vi "mainUI.vi"(8 "Error In":errorcluster, 10 "UI Data":T1, 11 "UDE Data":T14) -> (0 "Error Out":errorcluster)   [LabVIEW 2018]
uses:
  controls/uiUDE.ctl
  controls/uiData.ctl
  controls/pathCluster.ctl
  controls/shiftCluster.ctl
  controls/modelHomeCluster.ctl
  controls/hardwareSignalCluster.ctl
  controls/printedBarcodeCluster.ctl
  controls/scannedBarcode.ctl
  controls/reportCluster.ctl
  controls/modelSettingsCluster.ctl
  controls/LHndRH.ctl
  controls/ModelTableCluster.ctl
  controls/overrideCluster.ctl
  controls/countCluster.ctl
  Controller Module/src/controls/controllerData.ctl
  controls/mainAppElementsCluster.ctl
  Modbus Module/src/controls/modbusData.ctl
  controls/readRegisterModbusCluster.ctl
  Barcode Printer Module/src/controls/printData.ctl
  Barcode Scanner Module/src/controls/scanData.ctl
panel:
  out "Tab Control":enum32{"Home", "Report", "Settings"}(tab)
  out "TRACEABILITY GRAPH":cluster{"X":dbl, "Y":dbl}[](graph)
  out "PRODUCTION DATE":string
  out "SEQUENCE NUMBER":string
  out "PART NUMBER":string
  out "SUPPLIER CODE":string
  out "MODEL":string
  out "PRINTED BARCODE":cluster{"Value":string}
  out "SCANNED BARCODE":cluster{"Value":string}
  out "TOTAL":dbl
  out "NG":dbl
  out "OK":dbl
  out "SHIFT":string
  out "Scanner":bool
  out "Printer":bool
  out "Database":bool
  out "PLC":bool
  in  "Settings":bool
  in  "Report":bool
  in  "Stop":bool
  out "Application Name":string
  out "Result Table":string[][](table)
  out "Status":string
  out "Version No":string
  in  "Reprint":bool
  in  "TO DATE":timestamp format="%<%x %.3X>T"
  in  "Fetch":bool
  in  "Export":bool
  in  "FROM DATE":timestamp format="%<%x %.3X>T"
  out "Report Table":string[][](table)
  in  "Home":bool
  in  "NG":string
  in  "OK":string
  in  "SEQUENCE NUMBER":string
  in  "Override Button":bool
  in  "Load Button":bool
  in  "Home Button":bool
  in  "Delete Button":bool
  in  "Update Button":bool
  in  "Save Button":bool
  in  "PLC NUMBER":string
  in  "LH / RH":T10
  in  "SUPPLIER CODE":string
  in  "CUSTOMER PART NUMBER":string
  in  "SAVED MODEL":string(combo)
  out "Model Table":string[][](table)
  in  "MODEL":string
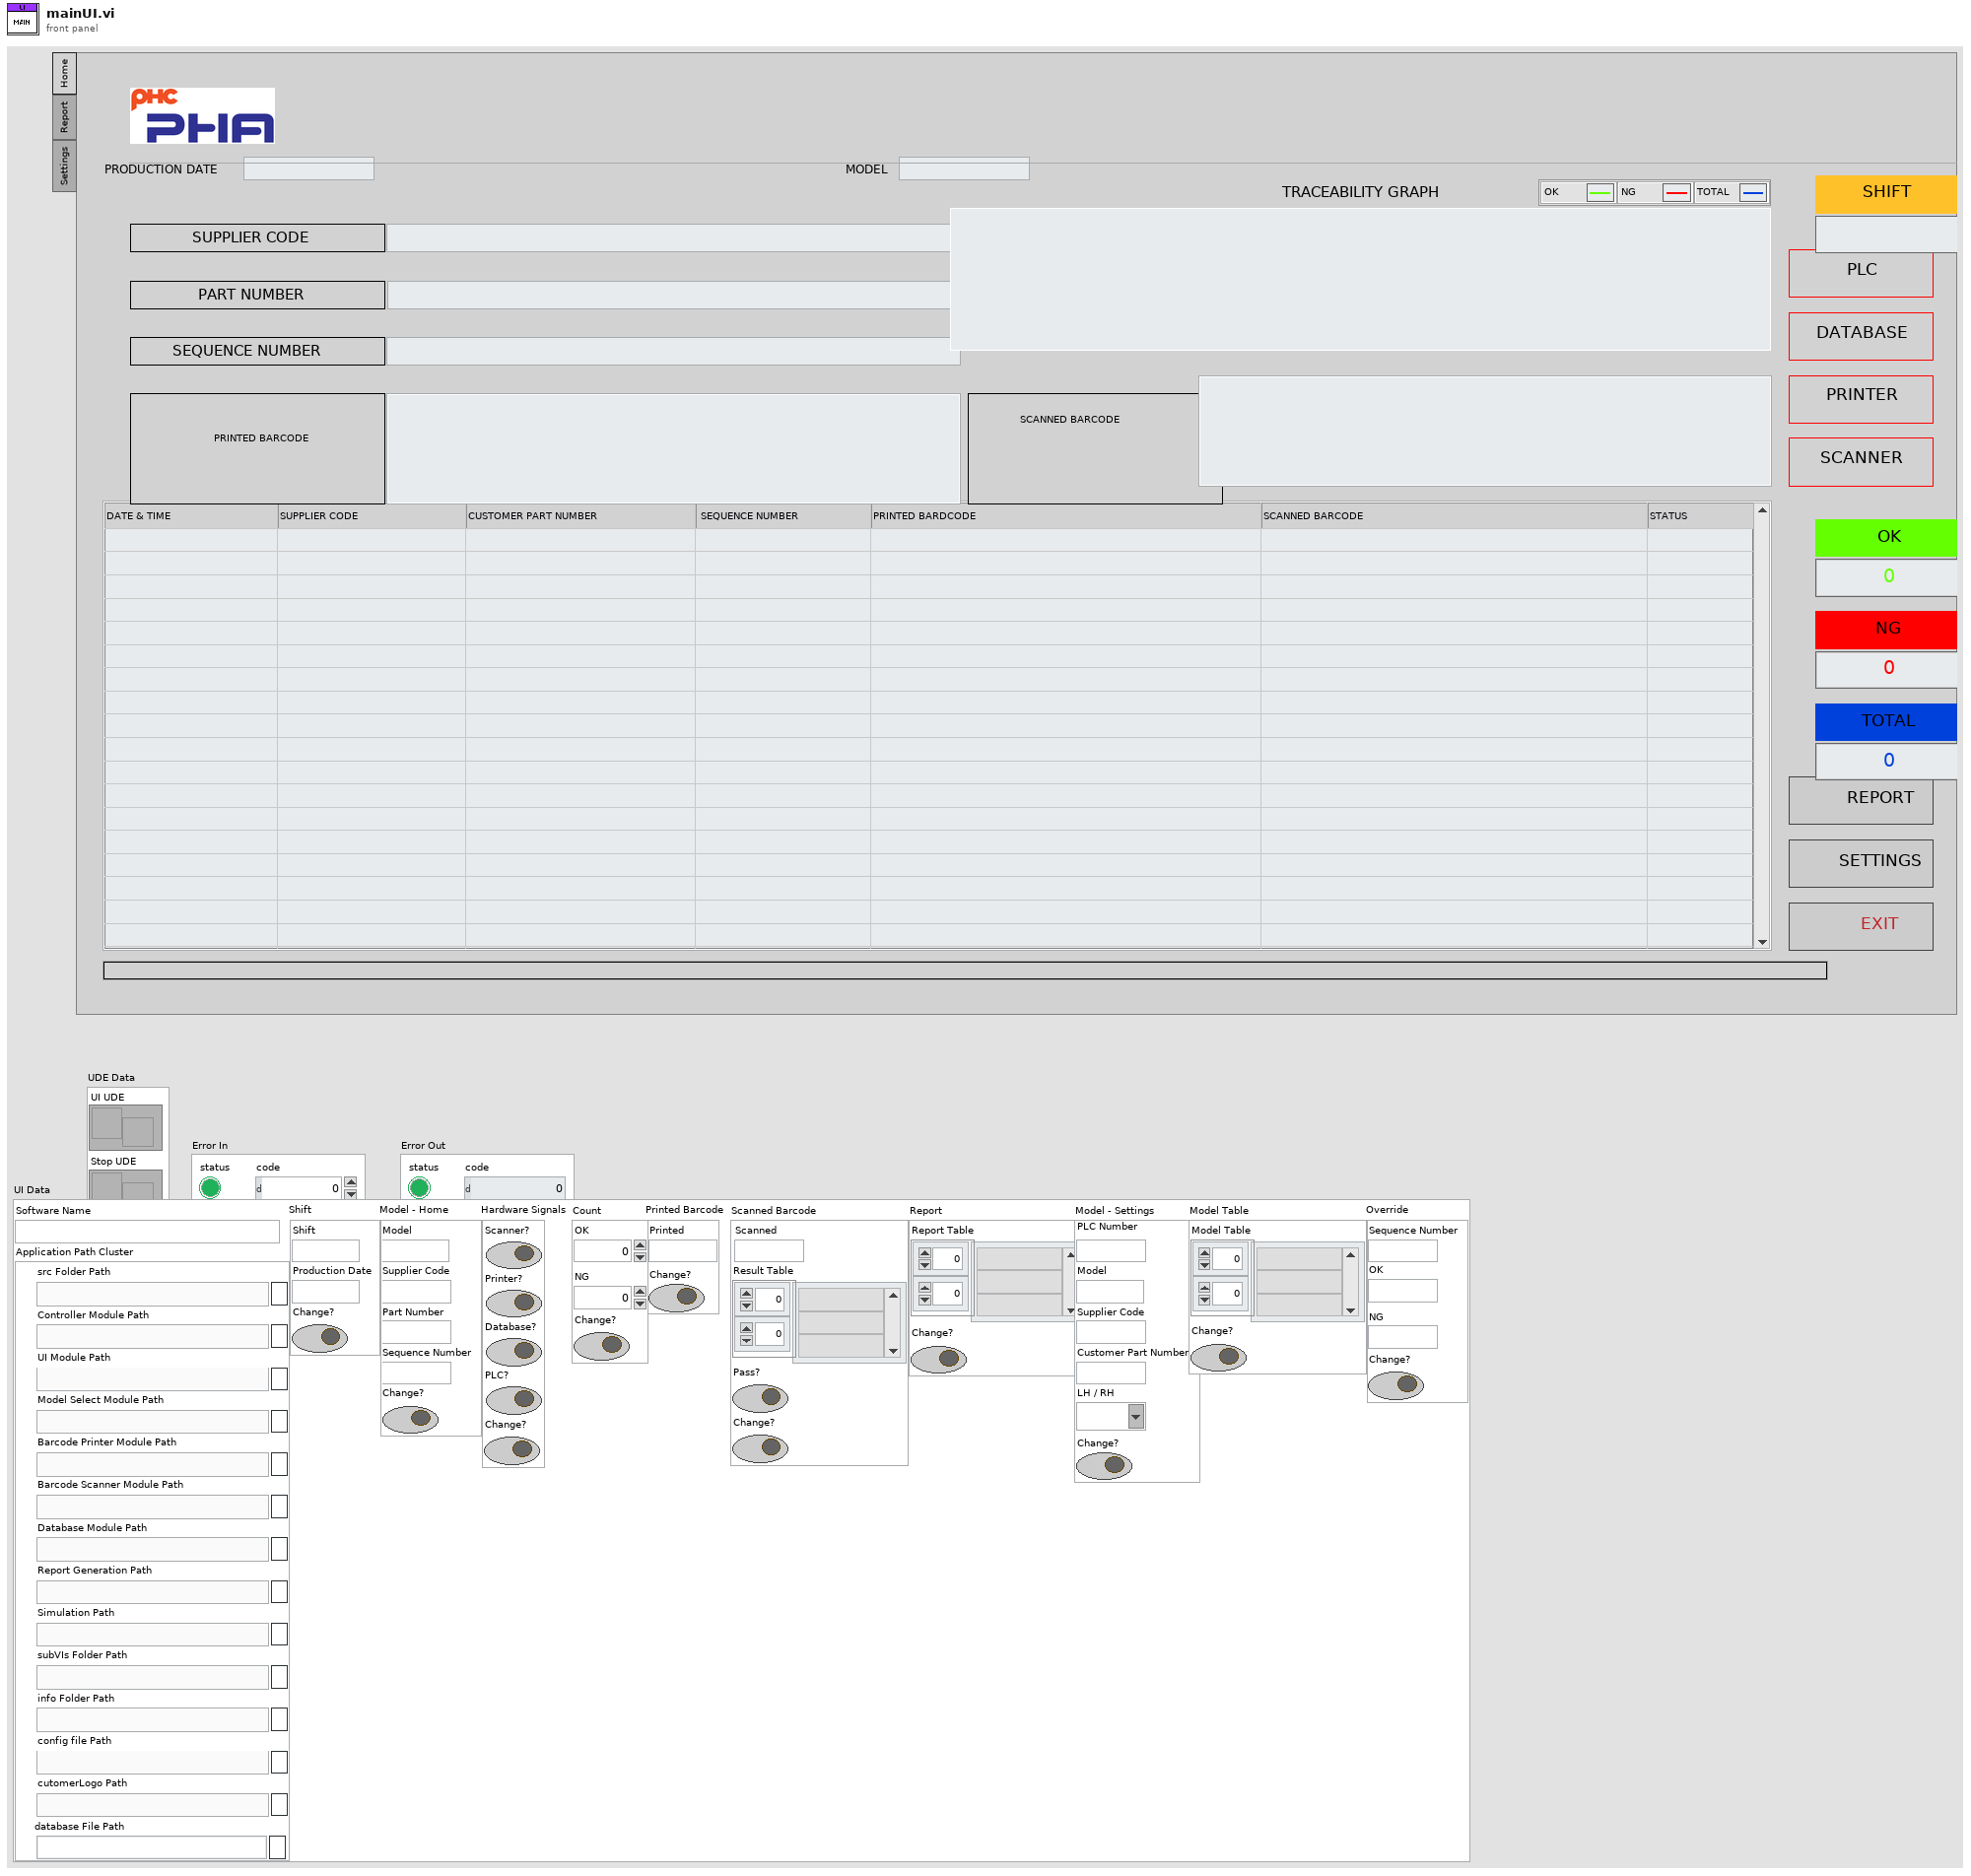
[diagram p1: front panel]
types:
  T1 = typedef "uiData.ctl" = cluster{"Software Name":string, "Application Path Cluster":T2, "Shift":T3, "Model - Home":T4, "Hardware Signals":T5, "Printed Barcode":T6, "Scanned Barcode":T7, "Report":T8, "Model - Settings":T9, "Model Table":T11, "Override":T12, "Count":T13}
  T2 = typedef "pathCluster.ctl" = cluster{"src Folder Path":path, "Controller Module Path":path, "UI Module Path":path, "Model Select Module Path":path, "Barcode Printer Module Path":path, "Barcode Scanner Module Path":path, "Database Module Path":path, "Report Generation Path":path, "Simulation Path":path, "subVIs Folder Path":path, "info Folder Path":path, "config file Path":path, "cutomerLogo Path":path, "database File Path":path}
  T3 = typedef "shiftCluster.ctl" = cluster{"Production Date":string, "Shift":string, "Change?":bool}
  T4 = typedef "modelHomeCluster.ctl" = cluster{"Model":string, "Supplier Code":string, "Part Number":string, "Sequence Number":string, "Change?":bool}
  T5 = typedef "hardwareSignalCluster.ctl" = cluster{"PLC?":bool, "Database?":bool, "Printer?":bool, "Scanner?":bool, "Change?":bool}
  T6 = typedef "printedBarcodeCluster.ctl" = cluster{"Printed":string, "Change?":bool}
  T7 = typedef "scannedBarcode.ctl" = cluster{"Scanned":string, "Result Table":string[][], "Change?":bool, "Pass?":bool}
  T8 = typedef "reportCluster.ctl" = cluster{"Report Table":string[][], "Change?":bool}
  T9 = typedef "modelSettingsCluster.ctl" = cluster{"Model":string, "Supplier Code":string, "Customer Part Number":string, "LH / RH":T10, "Change?":bool, "PLC Number":string}
  T10 = typedef "LHndRH.ctl" = string
  T11 = typedef "ModelTableCluster.ctl" = cluster{"Model Table":string[][], "Change?":bool}
  T12 = typedef "overrideCluster.ctl" = cluster{"Change?":bool, "Sequence Number":string, "OK":string, "NG":string}
  T13 = typedef "countCluster.ctl" = cluster{"Change?":bool, "OK":dbl, "NG":dbl}
  T14 = typedef "uiUDE.ctl" = cluster{"UI UDE":refnum<user-event>, "Stop UDE":refnum<user-event>, "Controller UDE":refnum<user-event>}
  T15 = typedef "mainAppElementsCluster.ctl" = cluster{"Application Name":refnum<vi>, "Tab Control":refnum<vi>, "Status":refnum<vi>, "Version No":refnum<vi>, "Result Table":refnum<vi>, "PLC":refnum<vi>, "Database":refnum<vi>, "Printer":refnum<vi>, "Scanner":refnum<vi>, "SHIFT":refnum<vi>, "OK":refnum<vi>, "NG":refnum<vi>, "TOTAL":refnum<vi>, "SCANNED BARCODE":refnum<vi>, " PRINTED BARCODE":refnum<vi>, "PART NUMBER":refnum<vi>, "PRODUCTION DATE":refnum<vi>, "SUPPLIER CODE":refnum<vi>, "SEQUENCE NUMBER":refnum<vi>, "MODEL":refnum<vi>, "Settings":refnum<vi>, "Report":refnum<vi>, "Report Table":refnum<vi>, "Home":refnum<vi>, "Export":refnum<vi>, "Fetch":refnum<vi>, "TO DATE":refnum<vi>, "FROM DATE":refnum<vi>, "Model Table":refnum<vi>, "Traceablity Graph":refnum<vi>, "Override Button":refnum<vi>, "Load Button":refnum<vi>, "Home Button-Setting":refnum<vi>, "Delete Button":refnum<vi>, "Update Button":refnum<vi>, "Save Button":refnum<vi>, "SEQUENCE NUMBER-Settings":refnum<vi>, "PLC NUMBER":refnum<vi>, "LH / RH":refnum<vi>, "SUPPLIER CODE-Setting":refnum<vi>, "CUSTOMER PART NUMBER-Setting":refnum<vi>, "MODEL-Setting":refnum<vi>, "SAVED MODEL":refnum<vi>, "NG-Settings":refnum<vi>, "OK-Settings":refnum<vi>}
  T16 = enum32{"Invalid", "Standard", "Closed", "Hidden", "Minimized", "Maximized"}
  T17 = enum32{"invalid app kind", "Development System", "Run Time System", "Student Edition", "Embedded LabVIEW", "Evaluation", "Custom"}
  T18 = typedef "controllerData.ctl" = cluster{"Actions":bool[], "UI Elements Cluster":T15, "Modbus Data":T19, "Print Data":T21, "Scan Data":T22}
  T19 = typedef "modbusData.ctl" = cluster{"IP Address":string, "Timeout":i32, "Port [502]":u16, "isSimulation?":bool, "Model Number":u16, "Read Modbus Register":T20, "Individual Address":u16[], "Model Changed?":bool, "Models Table":string[][], "Status?":bool}
  T20 = typedef "readRegisterModbusCluster.ctl" = cluster{"Starting Address":u16, "Number of Inputs":u16}
  T21 = typedef "printData.ctl" = cluster{"Print Button":bool, "VISA resource name":refnum<visa-resource-name>, "Status?":bool, "Scan?":bool}
  T22 = typedef "scanData.ctl" = cluster{"Scan Button":bool, "Status?":bool}
  T23 = cluster{"Core":cluster{"Current VI Reference":refnum<vi>, "Close Panel on Exit?":bool}, "UDE Data":T14, "Main App Cluster":T15, "UI Data":T1, "Actions":bool[]}
  T24 = cluster{"Current VI Reference":refnum<vi>, "Close Panel on Exit?":bool}
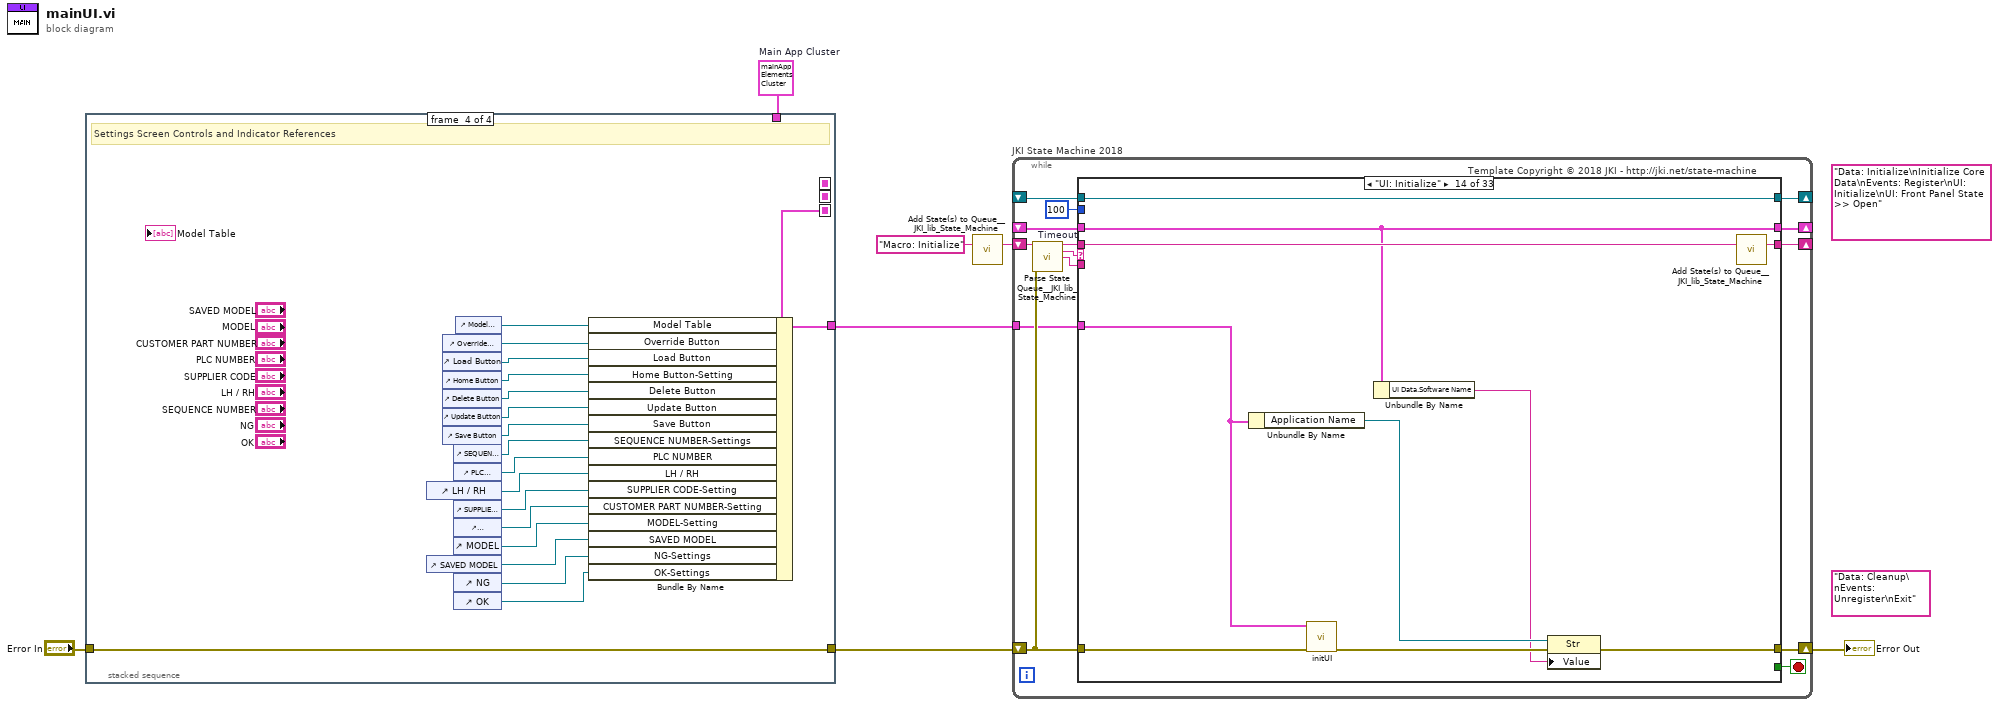
[diagram p0: block diagram]
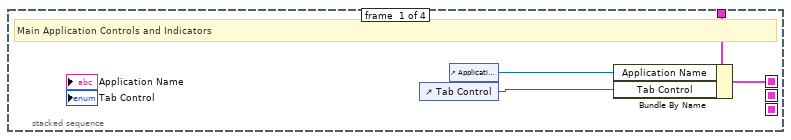
[diagram p2: hidden frame]
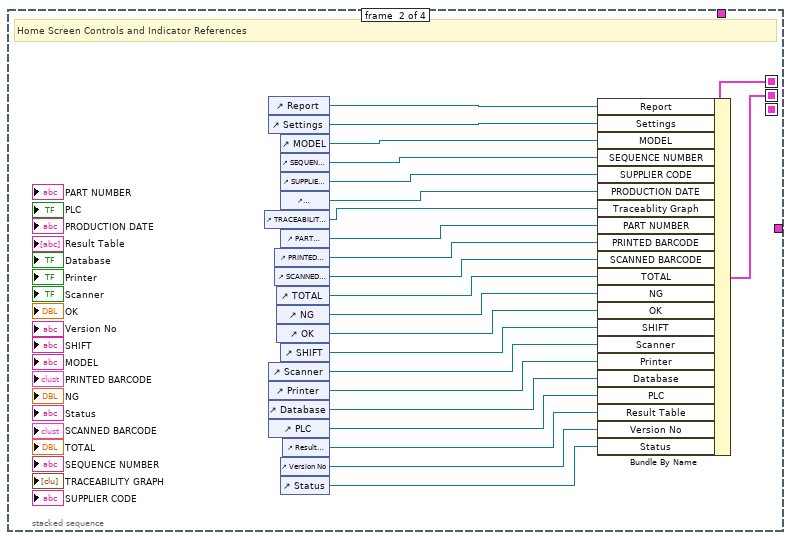
[diagram p3: hidden frame]
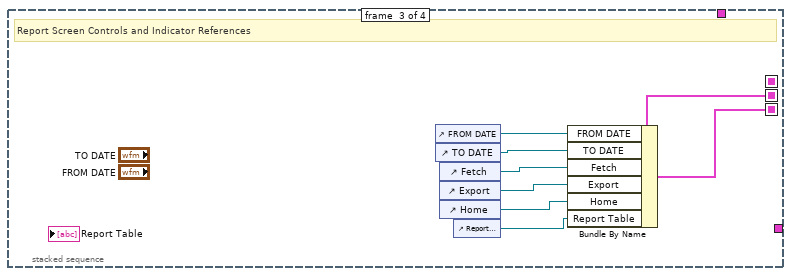
[diagram p4: hidden frame]
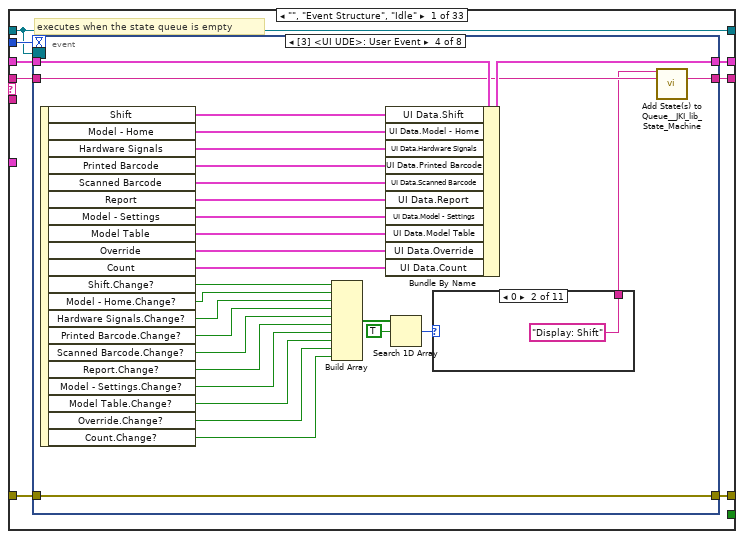
[diagram p5: hidden frame]
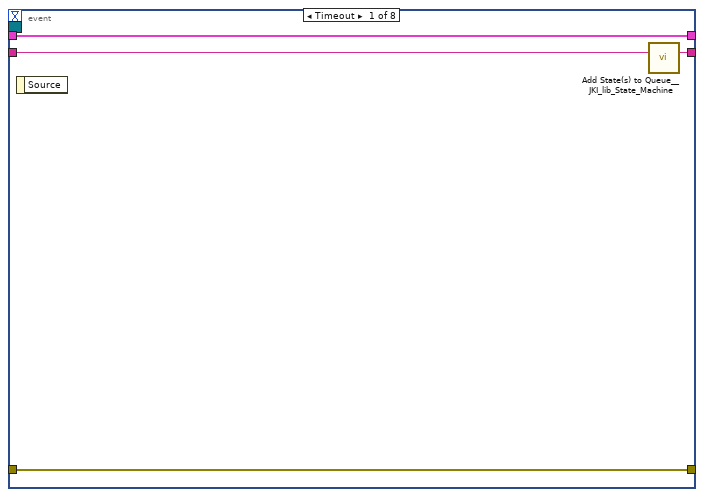
[diagram p6: hidden frame]
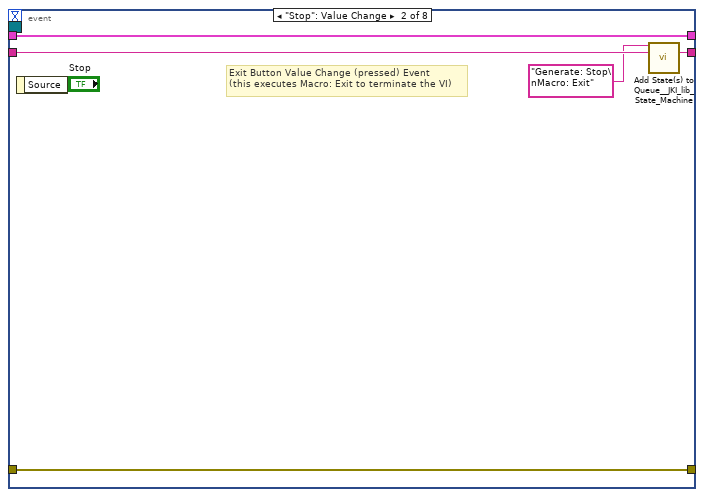
[diagram p7: hidden frame]
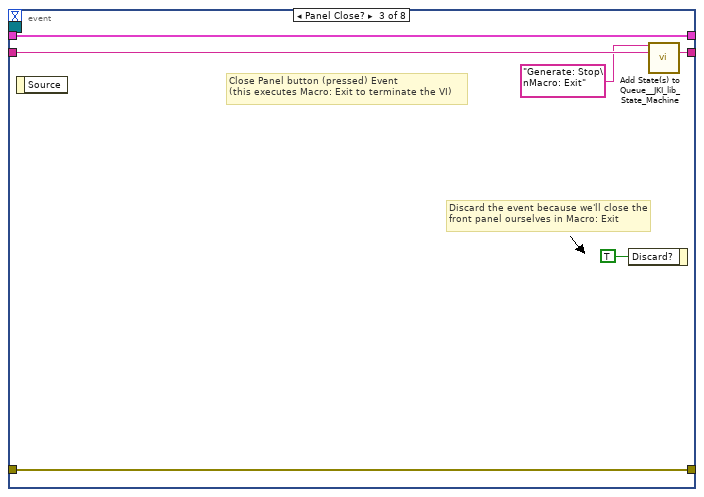
[diagram p8: hidden frame]
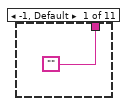
[diagram p9: hidden frame]
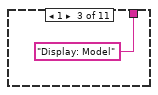
[diagram p10: hidden frame]
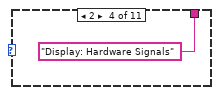
[diagram p11: hidden frame]
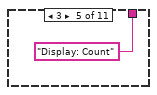
[diagram p12: hidden frame]
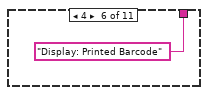
[diagram p13: hidden frame]
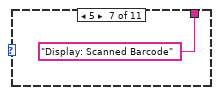
[diagram p14: hidden frame]
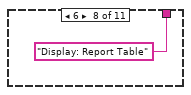
[diagram p15: hidden frame]
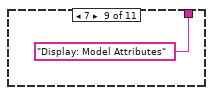
[diagram p16: hidden frame]
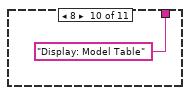
[diagram p17: hidden frame]
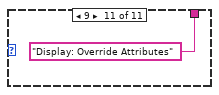
[diagram p18: hidden frame]
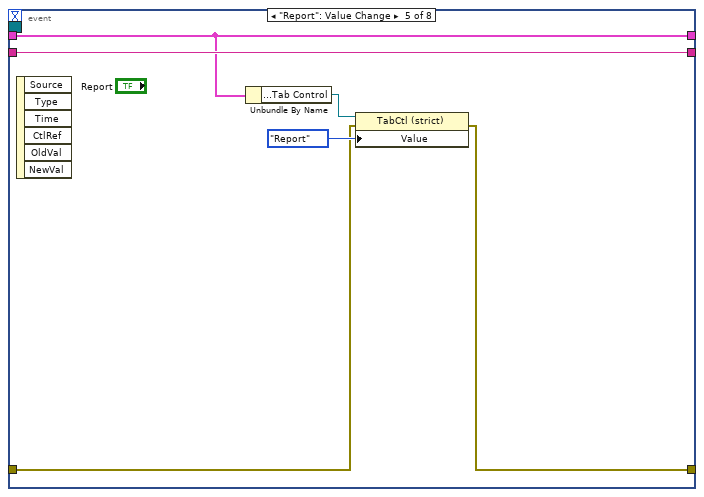
[diagram p19: hidden frame]
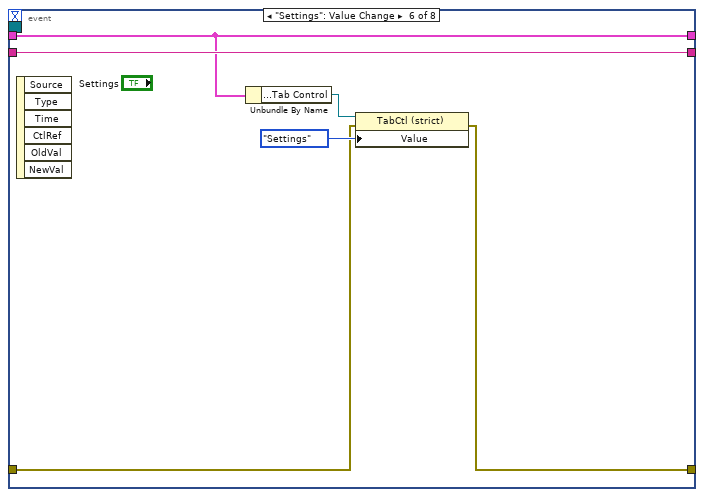
[diagram p20: hidden frame]
diagram:
  (unwired) "Data: Cleanup\nEvents: Unregister\nExit"
  (unwired) "Data: Initialize\nInitialize Core Data\nEvents: Register\nUI: Initialize\nUI: Front Panel State >> Open"
  w2 = T15 {"Application Name"=refnum, "Tab Control"=refnum, "Status"=refnum, "Version No"=refnum, "Result Table"=refnum, "PLC"=refnum, "Database"=refnum, "Printer"=refnum, "Scanner"=refnum, "SHIFT"=refnum, "OK"=refnum, "NG"=refnum, "TOTAL"=refnum, "SCANNED BARCODE"=refnum, " PRINTED BARCODE"=refnum, "PART NUMBER"=refnum, "PRODUCTION DATE"=refnum, "SUPPLIER CODE"=refnum, "SEQUENCE NUMBER"=refnum, "MODEL"=refnum, "Settings"=refnum, "Report"=refnum, "Report Table"=refnum, "Home"=refnum, "Export"=refnum, "Fetch"=refnum, "TO DATE"=refnum, "FROM DATE"=refnum, "Model Table"=refnum, "Traceablity Graph"=refnum, "Override Button"=refnum, "Load Button"=refnum, "Home Button-Setting"=refnum, "Delete Button"=refnum, "Update Button"=refnum, "Save Button"=refnum, "SEQUENCE NUMBER-Settings"=refnum, "PLC NUMBER"=refnum, "LH / RH"=refnum, "SUPPLIER CODE-Setting"=refnum, "CUSTOMER PART NUMBER-Setting"=refnum, "MODEL-Setting"=refnum, "SAVED MODEL"=refnum, "NG-Settings"=refnum, "OK-Settings"=refnum}  # Main App Cluster
  n1 = stacked-sequence {
    seq-local: [w9 _ _ _] -> [_ w14 _ _]
    seq-local: [_ w13 _ _] -> [_ _ w36 _]
    seq-local: [_ _ w35 _] -> [_ _ _ w61]
    tunnel: "Error In" -> [_ _ _ w58]
    tunnel: [_ _ _ w58] -> w4
    tunnel: w2 -> [w8 _ _ _]
    tunnel: [_ _ _ w60] -> w1
    frame #0 {
      # "Main Application Controls and Indicators"
      n2 = control-ref of="Tab Control"() -> (w10:refnum<vi>)
      n3 = control-ref of="Application Name"() -> (w11:refnum<vi>)
      n4 = Bundle By Name(cluster=w8, "Application Name"=w11, "Tab Control"=w10) -> (w9:T15)
    }
    frame #1 {
      # "Home Screen Controls and Indicator References"
      n5 = control-ref of="TRACEABILITY GRAPH"() -> (w12:refnum<vi>)
      n6 = control-ref of="Report"() -> (w34:refnum<vi>)
      n7 = control-ref of="Settings"() -> (w33:refnum<vi>)
      n8 = control-ref of="Scanner"() -> (w21:refnum<vi>)
      n9 = control-ref of="Printer"() -> (w20:refnum<vi>)
      n10 = control-ref of="Database"() -> (w19:refnum<vi>)
      n11 = control-ref of="PLC"() -> (w18:refnum<vi>)
      n12 = control-ref of="PRINTED BARCODE"() -> (w27:refnum<vi>)
      n13 = control-ref of="SCANNED BARCODE"() -> (w26:refnum<vi>)
      n14 = control-ref of="TOTAL"() -> (w25:refnum<vi>)
      n15 = control-ref of="NG"() -> (w24:refnum<vi>)
      n16 = control-ref of="OK"() -> (w23:refnum<vi>)
      n17 = control-ref of="MODEL"() -> (w32:refnum<vi>)
      n18 = control-ref of="SEQUENCE NUMBER"() -> (w31:refnum<vi>)
      n19 = control-ref of="SUPPLIER CODE"() -> (w30:refnum<vi>)
      n20 = control-ref of="PRODUCTION DATE"() -> (w29:refnum<vi>)
      n21 = control-ref of="PART NUMBER"() -> (w28:refnum<vi>)
      n22 = control-ref of="SHIFT"() -> (w22:refnum<vi>)
      n23 = control-ref of="Version No"() -> (w16:refnum<vi>)
      n24 = control-ref of="Status"() -> (w15:refnum<vi>)
      n25 = control-ref of="Result Table"() -> (w17:refnum<vi>)
      n26 = Bundle By Name(cluster=w14, "Report"=w34, "Settings"=w33, "MODEL"=w32, "SEQUENCE NUMBER"=w31, "SUPPLIER CODE"=w30, "PRODUCTION DATE"=w29, "Traceablity Graph"=w12, "PART NUMBER"=w28, "PRINTED BARCODE"=w27, "SCANNED BARCODE"=w26, "TOTAL"=w25, "NG"=w24, "OK"=w23, "SHIFT"=w22, "Scanner"=w21, "Printer"=w20, "Database"=w19, "PLC"=w18, "Result Table"=w17, "Version No"=w16, "Status"=w15) -> (w13:T15)
    }
    frame #2 {
      # "Report Screen Controls and Indicator References"
      n27 = control-ref of="FROM DATE"() -> (w42:refnum<vi>)
      n28 = control-ref of="TO DATE"() -> (w41:refnum<vi>)
      n29 = control-ref of="Fetch"() -> (w40:refnum<vi>)
      n30 = control-ref of="Export"() -> (w39:refnum<vi>)
      n31 = control-ref of="Home"() -> (w38:refnum<vi>)
      n32 = control-ref of="Report Table"() -> (w37:refnum<vi>)
      n33 = Bundle By Name(cluster=w36, "FROM DATE"=w42, "TO DATE"=w41, "Fetch"=w40, "Export"=w39, "Home"=w38, "Report Table"=w37) -> (w35:T15)
    }
    frame #3 {
      # "Settings Screen Controls and Indicator References"
      n34 = control-ref of="LH / RH"() -> (w49:refnum<vi>)
      n35 = control-ref of="SAVED MODEL"() -> (w45:refnum<vi>)
      n36 = control-ref of="Override Button"() -> (w57:refnum<vi>)
      n37 = control-ref of="Load Button"() -> (w56:refnum<vi>)
      n38 = control-ref of="Home Button"() -> (w55:refnum<vi>)
      n39 = control-ref of="Delete Button"() -> (w54:refnum<vi>)
      n40 = control-ref of="Update Button"() -> (w53:refnum<vi>)
      n41 = control-ref of="Save Button"() -> (w52:refnum<vi>)
      n42 = control-ref of="SEQUENCE NUMBER"() -> (w51:refnum<vi>)
      n43 = control-ref of="PLC NUMBER"() -> (w50:refnum<vi>)
      n44 = control-ref of="SUPPLIER CODE"() -> (w48:refnum<vi>)
      n45 = control-ref of="CUSTOMER PART NUMBER"() -> (w47:refnum<vi>)
      n46 = control-ref of="MODEL"() -> (w46:refnum<vi>)
      n47 = control-ref of="NG"() -> (w44:refnum<vi>)
      n48 = control-ref of="OK"() -> (w43:refnum<vi>)
      n49 = control-ref of="Model Table"() -> (w59:refnum<vi>)
      n50 = Bundle By Name(cluster=w61, "Model Table"=w59, "Override Button"=w57, "Load Button"=w56, "Home Button-Setting"=w55, "Delete Button"=w54, "Update Button"=w53, "Save Button"=w52, "SEQUENCE NUMBER-Settings"=w51, "PLC NUMBER"=w50, "LH / RH"=w49, "SUPPLIER CODE-Setting"=w48, "CUSTOMER PART NUMBER-Setting"=w47, "MODEL-Setting"=w46, "SAVED MODEL"=w45, "NG-Settings"=w44, "OK-Settings"=w43) -> (w60:T15)
    }
  }
  n51 = call <vilib>:"Add State(s) to Queue__JKI_lib_State_Machine.vi"("State(s) in (\"\")"="Macro: Initialize") -> ("States Out"=w7:string)  [unwired: 14 in]
  n52 = while "JKI State Machine 2018" {
    shift-right: [w68] -> _
    shift-left: _ -> [w67]
    shift-right: [w71] -> w3
    shift-left: w4 -> [w65]
    shift-right: [w70] -> _
    shift-left: w7 -> [w72]
    shift-right: [w64] -> _
    shift-left: _ -> [w63]
    tunnel: w1 -> [w62]
    stop <- w69 stop-if-true
    w66 = 100  # Timeout
    # "Template Copyright © 2018 JKI - http://jki.net/state-machine"
    n53 = call <vilib>:"Parse State Queue__JKI_lib_State_Machine.vi"("State Queue"=w72, "Error In (no error)"=w65) -> ("Remaining States"=w74:string, "Current State"=w75:string, "Arguments"=w73:string)  [unwired: 11 in]
    n54 = case shown="\"UI: Initialize\"" w75 {
      selector: w75 -> [_ _ w178 _ _ _ _ _ _ _ _ _ _ _ _ _ _ _ _ _ _ _ _ _ _ _ _ _ _ _ _ _ _]
      tunnel: w74 -> [w83 w176 w182 w202 w209 w215 w220 w230 w237 w242 w250 w256 w261 w271 w278 w290 w360 w366 w377 w382 w394 w412 w434 w449 w461 w484 w496 w517 w525 w540 w545 w555 w576]
      tunnel: w73 -> [_ _ _ _ _ _ _ _ _ _ _ _ _ _ w273 w284 _ _ _ _ _ _ _ _ _ _ _ _ _ _ _ _ _]
      tunnel: w67 -> [w81 w173 w180 w195 w206 w213 w217 _ w232 w239 w246 w254 w258 w267 w276 w286 w357 w363 w374 w379 w391 w409 w431 w446 w458 w481 w493 w514 w522 w537 w542 w548 w568]
      tunnel: [w80 w174 w184 w199 errorcluster {"status"=FALSE, "code"=0, "source"=""} ("error out") w212 w218 w227 w233 w240 w247 w251 w259 w263 w274 w287 w358 w364 w375 w380 w383 w403 w426 w441 w451 w480 w492 w511 w518 w531 w543 w551 w572] -> w71
      tunnel: w65 -> [w79 w174 w183 w199 w205 w212 w218 w227 w234 w240 w245 w252 w259 w268 w275 w288 w358 w364 w375 w380 w386 w397 w415 w439 w456 w463 w490 w506 w519 w532 w543 w552 w573]
      tunnel: [w82 w175 w181 w201 w208 w214 w219 w229 w236 w241 w249 w255 w260 w270 w277 w289 w359 w365 w376 w381 w393 w411 w433 w448 w460 w483 w495 w516 w524 w539 w544 w554 w575] -> w70
      tunnel: [_ _ _ _ _ TRUE _ _ _ _ _ _ _ _ _ _ _ _ _ _ _ _ _ _ _ _ _ _ _ _ _ _ _] -> w69
      tunnel: [w78 w173 w180 w200 w206 w213 w217 w228 w232 w239 w246 w254 w258 w267 w276 w286 w357 w363 w374 w379 w391 w409 w431 w446 w458 w481 w493 w514 w522 w537 w542 w547 w567] -> w68
      tunnel: w66 -> [w77 _ _ _ _ _ _ _ _ _ _ _ _ _ _ _ _ _ _ _ _ _ _ _ _ _ _ _ _ _ _ _ _]
      tunnel: [w76 w172 w177 w189 w203 w210 w216 w224 w231 w238 w248 w253 w257 w269 w272 w283 w356 w361 w367 w378 w392 w410 w432 w447 w459 w482 w494 w515 w523 w538 w541 w553 w574] -> w64
      tunnel: w63 -> [w76 w172 w177 w189 w203 w210 w216 w224 w231 w238 _ w253 w257 w269 w272 w283 w356 w361 w367 w378 w392 w410 w432 w447 w459 w482 w494 w515 w523 w538 w541 w553 w574]
      tunnel: w62 -> [_ _ _ _ _ _ _ w223 _ _ _ _ _ w266 _ _ _ _ _ _ _ _ _ _ _ _ _ _ _ _ _ _ _]
      frame "", "Event Structure", "Idle" {
        # "executes when the state queue is empty"
        n55 = event shown="[3] <UI UDE>: User Event" {
          selector: w76 -> [_ _ _ _ _ _ _ _]
          dyn-events: _ -> [_ _ _ _ _ _ _ _]
          timeout: w77 -> [_ _ _ _ _ _ _ _]
          tunnel: w83 -> [w87 w92 w98 w124 w144 w150 w156 w159]
          tunnel: [w86 w91 w97 w123 w144 w150 w156 w158] -> w82
          tunnel: w81 -> [w84 w89 w95 w126 w143 w149 w155 w170]
          tunnel: [w85 w90 w96 w127 w139 w145 w151 w171] -> w80
          tunnel: w79 -> [w85 w90 w96 w127 w140 w146 w152 w171]
          tunnel: [w84 w89 w95 w125 w143 w149 w155 w169] -> w78
          event Timeout {
            n56 = event-data() -> ()  [unwired: 1 in, 1 out]
            n57 = call <vilib>:"Add State(s) to Queue__JKI_lib_State_Machine.vi"("State(s) in (\"\")"=w87) -> ("States Out"=w86:string)  [unwired: 14 in]
          }
          event "Stop": Value Change {
            # "Exit Button Value Change (pressed) Event\n(this executes Macro: Exit to terminate the VI)"
            n58 = event-data() -> ()  [unwired: 1 in, 1 out]
            n59 = call <vilib>:"Add State(s) to Queue__JKI_lib_State_Machine.vi"("State(s) in Front (\"\")"="Generate: Stop\nMacro: Exit", "State(s) in (\"\")"=w92) -> ("States Out"=w91:string)  [unwired: 13 in]
          }
          event Panel Close? {
            # "Discard the event because we'll close the front panel ourselves in Macro: Exit"
            # "Close Panel button (pressed) Event\n(this executes Macro: Exit to terminate the VI)"
            n60 = event-data() -> ()  [unwired: 1 in, 1 out]
            n61 = event-data("Discard?"=TRUE) -> ()  [unwired: 1 in, 1 out]
            n62 = call <vilib>:"Add State(s) to Queue__JKI_lib_State_Machine.vi"("State(s) in Front (\"\")"="Generate: Stop\nMacro: Exit", "State(s) in (\"\")"=w98) -> ("States Out"=w97:string)  [unwired: 13 in]
          }
          event User Event {
            n63 = event-data() -> ("Shift"=w112:T3, "Model - Home"=w111:T4, "Hardware Signals"=w110:T5, "Printed Barcode"=w109:T6, "Scanned Barcode"=w108:T7, "Report"=w107:T8, "Model - Settings"=w106:T9, "Model Table"=w105:T11, "Override"=w104:T12, "Count"=w103:T13, "Shift.Change?"=w122:bool, "Model - Home.Change?"=w121:bool, "Hardware Signals.Change?"=w120:bool, "Printed Barcode.Change?"=w119:bool, "Scanned Barcode.Change?"=w118:bool, "Report.Change?"=w117:bool, "Model - Settings.Change?"=w116:bool, "Model Table.Change?"=w115:bool, "Override.Change?"=w114:bool, "Count.Change?"=w113:bool)  [unwired: 1 in]
            n64 = Build Array(w122, w121, w120, w119, w118, w117, w116, w115, w114, w113) -> (w101:bool[])
            n65 = Bundle By Name(cluster=w126, "UI Data.Shift"=w112, "UI Data.Model - Home"=w111, "UI Data.Hardware Signals"=w110, "UI Data.Printed Barcode"=w109, "UI Data.Scanned Barcode"=w108, "UI Data.Report"=w107, "UI Data.Model - Settings"=w106, "UI Data.Model Table"=w105, "UI Data.Override"=w104, "UI Data.Count"=w103) -> (w125:T23)
            n66 = Search 1D Array(1D array=w101, element=TRUE) -> (index of element=w102:i32)  [unwired: 1 in]
            n67 = case shown="0" w102 {
              tunnel: ["" "Display: Shift" ("State(s) in Front (\"\")") "Display: Model" ("State(s) in Front (\"\")") "Display: Hardware Signals" ("State(s) in Front (\"\")") "Display: Count" ("State(s) in Front (\"\")") "Display: Printed Barcode" ("State(s) in Front (\"\")") "Display: Scanned Barcode" ("State(s) in Front (\"\")") "Display: Report Table" ("State(s) in Front (\"\")") "Display: Model Attributes" ("State(s) in Front (\"\")") "Display: Model Table" ("State(s) in Front (\"\")") "Display: Override Attributes" ("State(s) in Front (\"\")")] -> w99
              frame -1, Default {
              }
              frame 0 {
              }
              frame 1 {
              }
              frame 2 {
              }
              frame 3 {
              }
              frame 4 {
              }
              frame 5 {
              }
              frame 6 {
              }
              frame 7 {
              }
              frame 8 {
              }
              frame 9 {
              }
            }
            n68 = call <vilib>:"Add State(s) to Queue__JKI_lib_State_Machine.vi"("State(s) in Front (\"\")"=w99, "State(s) in (\"\")"=w124) -> ("States Out"=w123:string)  [unwired: 13 in]
          }
          event "Report": Value Change {
            n69 = event-data() -> ()  [unwired: 1 in, 6 out]
            n70 = Unbundle By Name(w143) -> ("Main App Cluster.Tab Control"=w142:refnum<vi>)
            n71 = property class="TabCtl (strict)"(reference=w142, error in=w140, "Value"=enum32{"Home", "Report", "Settings"}."Report") -> (error out=w139:errorcluster)  [unwired: 1 out]
          }
          event "Settings": Value Change {
            n72 = event-data() -> ()  [unwired: 1 in, 6 out]
            n73 = Unbundle By Name(w149) -> ("Main App Cluster.Tab Control"=w148:refnum<vi>)
            n74 = property class="TabCtl (strict)"(reference=w148, error in=w146, "Value"=enum32{"Home", "Report", "Settings"}."Settings") -> (error out=w145:errorcluster)  [unwired: 1 out]
          }
          event "Home", "Home Button": Value Change {
            n75 = event-data() -> ()  [unwired: 1 in, 6 out]
            n76 = Unbundle By Name(w155) -> ("Main App Cluster.Tab Control"=w154:refnum<vi>)
            n77 = property class="TabCtl (strict)"(reference=w154, error in=w152, "Value"=enum32{"Home", "Report", "Settings"}."Home") -> (error out=w151:errorcluster)  [unwired: 1 out]
          }
          event "Fetch", "Export", "Reprint", "Save Button", "Update Button", "Delete Button", "Load Button", "Override Button": Value Change {
            n78 = event-data() -> ()  [unwired: 1 in, 6 out]
            n79 = Build Array("Fetch", "Export", "Reprint", "Save Button", "Update Button", "Delete Button", "Load Button", "Override Button") -> (w160:bool[])
            n80 = Bundle By Name(cluster=w170, "Actions"=w160) -> (w169:T23)
            n81 = call <vilib>:"Add State(s) to Queue__JKI_lib_State_Machine.vi"("State(s) in Front (\"\")"="Generate: Actions" ("State(s) in Front (\"\")"), "State(s) in (\"\")"=w159) -> ("States Out"=w158:string)  [unwired: 13 in]
          }
        }
      }
      frame "---------- Core ----------" {
        n82 = call <vilib>:"Add State(s) to Queue__JKI_lib_State_Machine.vi"("State(s) in (\"\")"=w176) -> ("States Out"=w175:string)  [unwired: 14 in]
      }
      frame Default {
        w187 = 42 items=["No error", "Argument error", "Memory is full", "Out of zone", "End of file", "File already open", "Generic file I/O error", "File not found", "File permission error", "Disk is full", "Duplicate path", "Too many files open", "System feature not enabled", "Resource file not found", "Cannot add resource", "Resource not found", "Image not found", "Image memory error", "Pen does not exist", "Config type invalid", "Config token not found", "Config parse error", "Config memory error", "Bad external code format", "Bad external code offset", "External code not present", "Null window", "Destroy window error", "Null menu", "Print aborted", "Bad print record", "Print driver error", "Windows error during printing", "Memory error during printing", "Print dialog error", "Generic print error", "Invalid device refnum", "Device not found", "Device parameter error", "Device unit error", "Cannot open device", "Device call aborted", "Generic error", "Cancelled by user", "Object ID too low", "Object ID too high", "Object not in heap", "Unknown heap", "Unknown object (invalid DefProc)", "Unknown object (DefProc not in table)", "Message out of range", "Invalid (null) method", "Unknown message", "Manager call not supported", "Bad address", "Network operation in progress", "Network operation timed out", "Connection is busy", "Network attribute not supported", "Network error", "Address in use", "System out of memory", "Connection aborted", "Connection refused", "Not connected", "Already connected", "Connection closed", "Initialization error (interapplication manager)", "Bad occurrence", "Wait on unbound occurrence handler", "Occurrence queue overflow", "Datalog type conflict", "Unused", "Unrecognized type (interapplication manager)", "Memory corrupt", "Failed to make temporary DLL", "Old CIN version", "Drag socket not found", "Failed to load drop-object", "Failed to register OLE object", "Failed to release OLE object", "Format specifier type mismatch", "Unknown format specifier", "Too few format specifiers", "Too many format specifiers", "Scan failed", "Newer CIN version", "Error converting to variant", "Runtime menu error", "Password tampered", "Variant attribute not found", "Incompatible variant data type", "Event data is not available", "Event Store is not present", "Occurrence is not found", "Event Queue is not created", "Event info is not available", "Refnum passed is NULL", "Error retrieving Class GUID", "Error retrieving CoClass GUID", "Error retrieving TypeLib GUID.", "Bad built application magic bytes.", "Specific driver is different from the specific driver associated with the Logical Name.", "There is no session opened to the class driver.", "Max Error", "MAX - Error with config objects", "MAX - Error loading configuration", "MAX - Group not supported"]
        # "Current State"
        # "Handle mistyped state name (developer tool)"
        n83 = Format Into String(format string="Software Exception: Unhandled State \"%s\"." ("message"), error in=w183, w178) -> (resulting string=w186:string, error out=w185:errorcluster)  [unwired: 1 in]
        n84 = call <vilib>:"Error Cluster From Error Code.vi"("show call chain? (False)"=TRUE, "error in (no error)"=w185, "error message (\"\")"=w186, "error code (0)"=w187) -> ("error out"=w184:errorcluster)  [unwired: 5 in]
        n85 = call <vilib>:"Add State(s) to Queue__JKI_lib_State_Machine.vi"("State(s) in (\"\")"=w182) -> ("States Out"=w181:string)  [unwired: 14 in]
      }
      frame "Initialize Core Data" {
        # "originally closed?"
        # "exe?"
        # "If panel starts closed or is an EXE, then close it when we exit"
        n86 = property class="VI"() -> ("FP.State"=w192:T16)  [unwired: 2 in, 2 out]
        n87 = property class="App"() -> ("App.Kind"=w198:T17)  [unwired: 2 in, 2 out]
        n88 = control-ref of="Current VI Reference"() -> (w193:refnum<vi>)
        n89 = Equal?(x=w192, y=T16."Closed" ("Front Panel Window:State")) -> (x = y?=w190:bool)
        n90 = Equal?(x=w198, y=T17."Run Time System" ("Application:Kind")) -> (x = y?=w196:bool)
        n91 = Or(x=w190, y=w196) -> (x .or. y?=w194:bool)
        n92 = Bundle By Name(cluster=w195, "Core.Current VI Reference"=w193, "Core.Close Panel on Exit?"=w194) -> (w200:T23)
        n93 = call <vilib>:"Add State(s) to Queue__JKI_lib_State_Machine.vi"("State(s) in (\"\")"=w202) -> ("States Out"=w201:string)  [unwired: 14 in]
      }
      frame "Error Handler" {
        # "Unhandled Error -- Display it"
        # "Clear error"
        n94 = call <vilib>:"General Error Handler.vi"("error in (no error)"=w205) -> ()  [unwired: 10 in, 5 out]
        n95 = call <vilib>:"Add State(s) to Queue__JKI_lib_State_Machine.vi"("State(s) in Front (\"\")"="/* Post Error States", "State(s) in (\"\")"=w209) -> ("States Out"=w208:string)  [unwired: 13 in]
      }
      frame "Exit" {
        n96 = call <vilib>:"Add State(s) to Queue__JKI_lib_State_Machine.vi"("State(s) in (\"\")"=w215) -> ("States Out"=w214:string)  [unwired: 14 in]
      }
      frame "---------- Data ----------" {
        n97 = call <vilib>:"Add State(s) to Queue__JKI_lib_State_Machine.vi"("State(s) in (\"\")"=w220) -> ("States Out"=w219:string)  [unwired: 14 in]
      }
      frame "Data: Initialize" {
        w222 = bool[] []  # Actions
        w226 = T24 {"Current VI Reference"=refnum, "Close Panel on Exit?"=FALSE}  # Core
        n98 = Bundle("Core"=w226, "UDE Data"="UDE Data", "Main App Cluster"=w223, "UI Data"="UI Data", "Actions"=w222) -> (w228:T23)  [unwired: 1 in]
        n99 = call <vilib>:"Add State(s) to Queue__JKI_lib_State_Machine.vi"("State(s) in (\"\")"=w230) -> ("States Out"=w229:string)  [unwired: 14 in]
      }
      frame "Data: Cleanup" {
        n100 = Unbundle By Name(w232) -> ("Core.Current VI Reference"=w235:refnum<vi>)
        n101 = Close Reference(reference=w235, error in (no error)=w234) -> (error out=w233:errorcluster)
        n102 = call <vilib>:"Add State(s) to Queue__JKI_lib_State_Machine.vi"("State(s) in (\"\")"=w237) -> ("States Out"=w236:string)  [unwired: 14 in]
      }
      frame "---------- Events ----------" {
        n103 = call <vilib>:"Add State(s) to Queue__JKI_lib_State_Machine.vi"("State(s) in (\"\")"=w242) -> ("States Out"=w241:string)  [unwired: 14 in]
      }
      frame "Events: Register" {
        n104 = Unbundle By Name(w246) -> ("UDE Data.UI UDE"=w244:refnum<user-event>, "UDE Data.Stop UDE"=w243:refnum<user-event>)
        n105 = register-events(error in=w245, w244, w243) -> (reference out=w248:refnum<event-registration>, error out=w247:errorcluster)  [unwired: 1 in]
        n106 = call <vilib>:"Add State(s) to Queue__JKI_lib_State_Machine.vi"("State(s) in (\"\")"=w250) -> ("States Out"=w249:string)  [unwired: 14 in]
      }
      frame "Events: Unregister" {
        n107 = Unregister For Events(event registration refnum=w253, error in=w252) -> (error out=w251:errorcluster)
        n108 = call <vilib>:"Add State(s) to Queue__JKI_lib_State_Machine.vi"("State(s) in (\"\")"=w256) -> ("States Out"=w255:string)  [unwired: 14 in]
      }
      frame "---------- UI ----------" {
        n109 = call <vilib>:"Add State(s) to Queue__JKI_lib_State_Machine.vi"("State(s) in (\"\")"=w261) -> ("States Out"=w260:string)  [unwired: 14 in]
      }
      frame "UI: Initialize" {
        n110 = Unbundle By Name(w266) -> ("Application Name"=w265:refnum<vi>)
        n111 = call "initUI.vi"("Error In"=w268, "UI Elements Cluster"=w266) -> ("Error Out"=w264:errorcluster)  [unwired: 9 in]
        n112 = Unbundle By Name(w267) -> ("UI Data.Software Name"=w262:string)
        n113 = property class="Str"(reference=w265, error in=w264, "Value"=w262) -> (error out=w263:errorcluster)  [unwired: 1 out]
        n114 = call <vilib>:"Add State(s) to Queue__JKI_lib_State_Machine.vi"("State(s) in (\"\")"=w271) -> ("States Out"=w270:string)  [unwired: 14 in]
      }
      frame "UI: Cursor Set" {
        # "Argument"
        n115 = case shown="\"Idle\", Default" w273 {
          tunnel: w275 -> [w280 w282]
          tunnel: [w279 w281] -> w274
          frame "Idle", Default {
            n116 = call <vilib>:"Unset Busy.vi"("error in (no error)"=w280) -> ("error out"=w279:errorcluster)  [unwired: 10 in]
          }
          frame "Busy" {
            n117 = call <vilib>:"Set Busy.vi"("error in (no error)"=w282) -> ("error out"=w281:errorcluster)  [unwired: 9 in, 1 out]
          }
        }
        n118 = call <vilib>:"Add State(s) to Queue__JKI_lib_State_Machine.vi"("State(s) in (\"\")"=w278) -> ("States Out"=w277:string)  [unwired: 14 in]
      }
      frame "UI: Front Panel State" {
        # "Argument"
        n119 = Unbundle By Name(w286) -> ("Core.Current VI Reference"=w285:refnum<vi>)
        n120 = case shown="\"Open\", \"Standard\", Default" w284 {
          tunnel: w288 -> [w296 w311 w322 w335 w348]
          tunnel: [w298 w312 w324 w337 w350] -> w287
          tunnel: w285 -> [w297 w309 w323 w336 w349]
          frame "Open", "Standard", Default {
            w291 = T16."Standard" ("State")
            n121 = property class="VI"(reference=w297, error in=w296) -> (reference out=w294:refnum<vi>, error out=w295:errorcluster, "FP.State"=w293:T16)
            n122 = Not Equal?(x=w293, y=w291) -> (x != y?=w292:bool)
            n123 = case shown="True" w292 {
              tunnel: [w302 w304] -> w298
              tunnel: w295 -> [w301 w304]
              tunnel: w294 -> [w300 _]
              tunnel: w291 -> [w299 _]
              frame True {
                n124 = invoke class="VI" method="FP.Open"(reference=w300, error in=w301, "Activate"=TRUE, "State"=w299) -> (error out=w302:errorcluster)  [unwired: 1 in, 4 out]
              }
              frame False {
              }
            }
          }
          frame "Close", "Closed" {
            n125 = property class="VI"(reference=w309, error in=w311) -> (reference out=w308:refnum<vi>, error out=w310:errorcluster, "FP.State"=w306:T16)
            n126 = Not Equal?(x=w306, y=T16."Closed" ("Front Panel Window:State")) -> (x != y?=w305:bool)
            n127 = case shown="True" w305 {
              tunnel: [w313 w316] -> w312
              tunnel: w310 -> [w313 w315]
              tunnel: w308 -> [_ w314]
              frame False {
              }
              frame True {
                n128 = invoke class="VI" method="FP.Close"(reference=w314, error in=w315) -> (error out=w316:errorcluster)  [unwired: 1 in, 2 out]
              }
            }
          }
          frame "Hidden", "Hide" {
            w317 = T16."Hidden" ("State")
            n129 = property class="VI"(reference=w323, error in=w322) -> (reference out=w320:refnum<vi>, error out=w321:errorcluster, "FP.State"=w319:T16)
            n130 = Not Equal?(x=w319, y=w317) -> (x != y?=w318:bool)
            n131 = case shown="True" w318 {
              tunnel: [w328 w329] -> w324
              tunnel: w321 -> [w327 w329]
              tunnel: w320 -> [w326 _]
              tunnel: w317 -> [w325 _]
              frame True {
                n132 = invoke class="VI" method="FP.Open"(reference=w326, error in=w327, "State"=w325) -> (error out=w328:errorcluster)  [unwired: 2 in, 4 out]
              }
              frame False {
              }
            }
          }
          frame "Minimize", "Minimized" {
            w330 = T16."Minimized" ("State")
            n133 = property class="VI"(reference=w336, error in=w335) -> (reference out=w333:refnum<vi>, error out=w334:errorcluster, "FP.State"=w332:T16)
            n134 = Not Equal?(x=w332, y=w330) -> (x != y?=w331:bool)
            n135 = case shown="True" w331 {
              tunnel: [w341 w342] -> w337
              tunnel: w334 -> [w340 w342]
              tunnel: w333 -> [w339 _]
              tunnel: w330 -> [w338 _]
              frame True {
                n136 = invoke class="VI" method="FP.Open"(reference=w339, error in=w340, "State"=w338) -> (error out=w341:errorcluster)  [unwired: 2 in, 4 out]
              }
              frame False {
              }
            }
          }
          frame "Maximize", "Maximized" {
            w343 = T16."Maximized" ("State")
            n137 = property class="VI"(reference=w349, error in=w348) -> (reference out=w346:refnum<vi>, error out=w347:errorcluster, "FP.State"=w345:T16)
            n138 = Not Equal?(x=w345, y=w343) -> (x != y?=w344:bool)
            n139 = case shown="True" w344 {
              tunnel: [w354 w355] -> w350
              tunnel: w347 -> [w353 w355]
              tunnel: w346 -> [w352 _]
              tunnel: w343 -> [w351 _]
              frame True {
                n140 = invoke class="VI" method="FP.Open"(reference=w352, error in=w353, "State"=w351) -> (error out=w354:errorcluster)  [unwired: 2 in, 4 out]
              }
              frame False {
              }
            }
          }
        }
        n141 = call <vilib>:"Add State(s) to Queue__JKI_lib_State_Machine.vi"("State(s) in (\"\")"=w290) -> ("States Out"=w289:string)  [unwired: 14 in]
      }
      frame "---------- Macro ----------" {
        n142 = call <vilib>:"Add State(s) to Queue__JKI_lib_State_Machine.vi"("State(s) in (\"\")"=w360) -> ("States Out"=w359:string)  [unwired: 14 in]
      }
      frame "Macro: Initialize" {
        n143 = call <vilib>:"Add State(s) to Queue__JKI_lib_State_Machine.vi"("State(s) in Front (\"\")"="Data: Initialize\nInitialize Core Data\nEvents: Register\nUI: Initialize\nUI: Front Panel State >> Open", "State(s) in (\"\")"=w366) -> ("States Out"=w365:string)  [unwired: 13 in]
      }
      frame "Macro: Exit" {
        n144 = Unbundle By Name(w374) -> ("Core.Close Panel on Exit?"=w373:bool)
        n145 = Select(t="UI: Front Panel State >> Close", s=w373, f="") -> (s? t:f=w370:string)
        n146 = call <vilib>:"Add State(s) to Queue__JKI_lib_State_Machine.vi"("State(s) in (\"\")"=w370, "State(s) at Back (\"\")"="Data: Cleanup\nEvents: Unregister\nExit") -> ("States Out"=w368:string)  [unwired: 13 in]
        n147 = call <vilib>:"Add State(s) to Queue__JKI_lib_State_Machine.vi"("State(s) in Front (\"\")"=w368, "State(s) in (\"\")"=w377) -> ("States Out"=w376:string)  [unwired: 13 in]
      }
      frame "---------- Display ----------" {
        n148 = call <vilib>:"Add State(s) to Queue__JKI_lib_State_Machine.vi"("State(s) in (\"\")"=w382) -> ("States Out"=w381:string)  [unwired: 14 in]
      }
      frame "Display: Shift" {
        n149 = Unbundle By Name(w391) -> ("Main App Cluster.SHIFT"=w390:refnum<vi>, "UI Data.Shift.Shift"=w389:string, "Main App Cluster.PRODUCTION DATE"=w388:refnum<vi>, "UI Data.Shift.Production Date"=w387:string)
        n150 = property class="Str"(reference=w390, error in=w386, "Value"=w389) -> (error out=w385:errorcluster)  [unwired: 1 out]
        n151 = property class="Str"(reference=w388, error in=w386, "Value"=w387) -> (error out=w384:errorcluster)  [unwired: 1 out]
        n152 = Merge Errors(w385, w384) -> (w383:errorcluster)
        n153 = call <vilib>:"Add State(s) to Queue__JKI_lib_State_Machine.vi"("State(s) in (\"\")"=w394) -> ("States Out"=w393:string)  [unwired: 14 in]
      }
      frame "Display: Model" {
        n154 = Unbundle By Name(w409) -> ("Main App Cluster.MODEL"=w408:refnum<vi>, "UI Data.Model - Home.Model"=w402:string, "Main App Cluster.SUPPLIER CODE"=w407:refnum<vi>, "UI Data.Model - Home.Supplier Code"=w406:string, "Main App Cluster.PART NUMBER"=w401:refnum<vi>, "UI Data.Model - Home.Part Number"=w400:string, "Main App Cluster.SEQUENCE NUMBER"=w399:refnum<vi>, "UI Data.Model - Home.Sequence Number"=w398:string)
        n155 = property class="Str"(reference=w408, error in=w397, "Value"=w402) -> (error out=w405:errorcluster)  [unwired: 1 out]
        n156 = property class="Str"(reference=w407, error in=w397, "Value"=w406) -> (error out=w404:errorcluster)  [unwired: 1 out]
        n157 = property class="Str"(reference=w401, error in=w397, "Value"=w400) -> (error out=w396:errorcluster)  [unwired: 1 out]
        n158 = property class="Str"(reference=w399, error in=w397, "Value"=w398) -> (error out=w395:errorcluster)  [unwired: 1 out]
        n159 = Merge Errors(w405, w404, w396, w395) -> (w403:errorcluster)
        n160 = call <vilib>:"Add State(s) to Queue__JKI_lib_State_Machine.vi"("State(s) in (\"\")"=w412) -> ("States Out"=w411:string)  [unwired: 14 in]
      }
      frame "Display: Hardware Signals" {
        n161 = Unbundle By Name(w431) -> ("Main App Cluster.PLC"=w430:refnum<vi>, "UI Data.Hardware Signals.PLC?"=w425:bool, "Main App Cluster.Database"=w429:refnum<vi>, "UI Data.Hardware Signals.Database?"=w423:bool, "Main App Cluster.Printer"=w421:refnum<vi>, "UI Data.Hardware Signals.Printer?"=w419:bool, "Main App Cluster.Scanner"=w420:refnum<vi>, "UI Data.Hardware Signals.Scanner?"=w418:bool)
        n162 = To Variant(anything=w425) -> (Variant=w424:variant)
        n163 = To Variant(anything=w423) -> (Variant=w422:variant)
        n164 = To Variant(anything=w419) -> (Variant=w417:variant)
        n165 = To Variant(anything=w418) -> (Variant=w416:variant)
        n166 = property class="Bool"(reference=w430, error in=w415, "Value"=w424) -> (error out=w428:errorcluster)  [unwired: 1 out]
        n167 = property class="Bool"(reference=w429, error in=w415, "Value"=w422) -> (error out=w427:errorcluster)  [unwired: 1 out]
        n168 = property class="Bool"(reference=w421, error in=w415, "Value"=w417) -> (error out=w414:errorcluster)  [unwired: 1 out]
        n169 = property class="Bool"(reference=w420, error in=w415, "Value"=w416) -> (error out=w413:errorcluster)  [unwired: 1 out]
        n170 = Merge Errors(w428, w427, w414, w413) -> (w426:errorcluster)
        n171 = call <vilib>:"Add State(s) to Queue__JKI_lib_State_Machine.vi"("State(s) in (\"\")"=w434) -> ("States Out"=w433:string)  [unwired: 14 in]
      }
      frame "Display: Count" {
        n172 = Unbundle By Name(w446) -> ("Main App Cluster.OK"=w445:refnum<vi>, "UI Data.Count.OK"=w436:dbl, "Main App Cluster.NG"=w444:refnum<vi>, "UI Data.Count.NG"=w435:dbl, "Main App Cluster.TOTAL"=w440:refnum<vi>)
        n173 = Add(x=w436, y=w435) -> (x+y=w437:dbl)
        n174 = property class="DigNum (strict)"(reference=w445, error in=w439, "Value"=w436) -> (error out=w443:errorcluster)  [unwired: 1 out]
        n175 = property class="DigNum (strict)"(reference=w444, error in=w439, "Value"=w435) -> (error out=w442:errorcluster)  [unwired: 1 out]
        n176 = property class="DigNum (strict)"(reference=w440, error in=w439, "Value"=w437) -> (error out=w438:errorcluster)  [unwired: 1 out]
        n177 = Merge Errors(w443, w442, w438) -> (w441:errorcluster)
        n178 = call <vilib>:"Add State(s) to Queue__JKI_lib_State_Machine.vi"("State(s) in (\"\")"=w449) -> ("States Out"=w448:string)  [unwired: 14 in]
      }
      frame "Display: Printed Barcode" {
        n179 = Unbundle By Name(w458) -> ("Main App Cluster.PRINTED BARCODE"=w457:refnum<vi>, "UI Data.Printed Barcode.Printed"=w454:string)
        n180 = property class="Clust (strict)"(reference=w457, error in=w456) -> (reference out=w453:refnum<vi>, error out=w452:errorcluster, "Value"=w455:cluster{"Value":string})
        n181 = Bundle By Name(cluster=w455, "Value"=w454) -> (w450:cluster{"Value":string})
        n182 = property class="Clust (strict)"(reference=w453, error in=w452, "Value"=w450) -> (error out=w451:errorcluster)  [unwired: 1 out]
        n183 = call <vilib>:"Add State(s) to Queue__JKI_lib_State_Machine.vi"("State(s) in (\"\")"=w461) -> ("States Out"=w460:string)  [unwired: 14 in]
      }
      frame "Display: Scanned Barcode" {
        n184 = Unbundle By Name(w481) -> ("Main App Cluster.SCANNED BARCODE"=w476:refnum<vi>, "UI Data.Scanned Barcode.Scanned"=w471:string, "Main App Cluster.PRINTED BARCODE"=w475:refnum<vi>, "UI Data.Scanned Barcode.Pass?"=w466:bool, "Main App Cluster.Result Table"=w465:refnum<vi>, "UI Data.Scanned Barcode.Result Table"=w464:string[][])
        n185 = Build Array(w476, w475) -> (w477:refnum<vi>[])
        n186 = Select(t=u32 6618880 ("Color"), s=w466, f=u32 16711680) -> (s? t:f=w478:u32)
        n187 = property class="Clust (strict)"(reference=w476, error in=w463) -> (reference out=w469:refnum<vi>, error out=w470:errorcluster, "Value"=w472:cluster{"Value":string})
        n188 = for {
          tunnel: w478 -> [w488]
          tunnel: w477 -> [w487] mode=indexing
          shift-right: [w486] -> w473
          shift-left: w463 -> [w485]
          n189 = property class="Clust (strict)"(reference=w487, error in=w485, "Color"=w488) -> (error out=w486:errorcluster)  [unwired: 1 out]
        }
        n190 = property class="Tbl (strict)"(reference=w465, error in=w463, "Value"=w464) -> (error out=w462:errorcluster)  [unwired: 1 out]
        n191 = Bundle By Name(cluster=w472, "Value"=w471) -> (w468:cluster{"Value":string})
        n192 = property class="Clust (strict)"(reference=w469, error in=w470, "Value"=w468) -> (error out=w467:errorcluster)  [unwired: 1 out]
        n193 = Merge Errors(w467, w473, w462) -> (w480:errorcluster)
        n194 = call <vilib>:"Add State(s) to Queue__JKI_lib_State_Machine.vi"("State(s) in (\"\")"=w484) -> ("States Out"=w483:string)  [unwired: 14 in]
      }
      frame "Display: Report Table" {
        n195 = Unbundle By Name(w493) -> ("Main App Cluster.Report Table"=w491:refnum<vi>, "UI Data.Report.Report Table"=w489:string[][])
        n196 = property class="Tbl (strict)"(reference=w491, error in=w490, "Value"=w489) -> (error out=w492:errorcluster)  [unwired: 1 out]
        n197 = call <vilib>:"Add State(s) to Queue__JKI_lib_State_Machine.vi"("State(s) in (\"\")"=w496) -> ("States Out"=w495:string)  [unwired: 14 in]
      }
      frame "Display: Model Attributes" {
        n198 = Unbundle By Name(w514) -> ("Main App Cluster.PLC NUMBER"=w512:refnum<vi>, "UI Data.Model - Settings.PLC Number"=w501:string, "Main App Cluster.MODEL-Setting"=w510:refnum<vi>, "UI Data.Model - Settings.Model"=w500:string, "Main App Cluster.LH / RH"=w509:refnum<vi>, "UI Data.Model - Settings.LH / RH"=w499:T10, "Main App Cluster.SUPPLIER CODE-Setting"=w508:refnum<vi>, "UI Data.Model - Settings.Supplier Code"=w498:string, "Main App Cluster.CUSTOMER PART NUMBER-Setting"=w507:refnum<vi>, "UI Data.Model - Settings.Customer Part Number"=w497:string)
        n199 = property class="CmbBox (strict)"(reference=w509, error in=w506, "Value"=w499) -> (error out=w504:errorcluster)  [unwired: 1 out]
        n200 = property class="Str"(reference=w512, error in=w506, "Value"=w501) -> (error out=w513:errorcluster)  [unwired: 1 out]
        n201 = property class="Str"(reference=w510, error in=w506, "Value"=w500) -> (error out=w505:errorcluster)  [unwired: 1 out]
        n202 = property class="Str"(reference=w508, error in=w506, "Value"=w498) -> (error out=w503:errorcluster)  [unwired: 1 out]
        n203 = property class="Str"(reference=w507, error in=w506, "Value"=w497) -> (error out=w502:errorcluster)  [unwired: 1 out]
        n204 = Merge Errors(w513, w505, w504, w503, w502) -> (w511:errorcluster)
        n205 = call <vilib>:"Add State(s) to Queue__JKI_lib_State_Machine.vi"("State(s) in (\"\")"=w517) -> ("States Out"=w516:string)  [unwired: 14 in]
      }
      frame "Display: Model Table" {
        n206 = Unbundle By Name(w522) -> ("Main App Cluster.Model Table"=w520:refnum<vi>, "UI Data.Model Table.Model Table"=w521:string[][])
        n207 = property class="Tbl (strict)"(reference=w520, error in=w519, "Value"=w521) -> (error out=w518:errorcluster)  [unwired: 1 out]
        n208 = call <vilib>:"Add State(s) to Queue__JKI_lib_State_Machine.vi"("State(s) in (\"\")"=w525) -> ("States Out"=w524:string)  [unwired: 14 in]
      }
      frame "Display: Override Attributes" {
        n209 = Unbundle By Name(w537) -> ("Main App Cluster.SEQUENCE NUMBER-Settings"=w536:refnum<vi>, "UI Data.Override.Sequence Number"=w526:string, "Main App Cluster.OK-Settings"=w534:refnum<vi>, "UI Data.Override.OK"=w528:string, "Main App Cluster.NG-Settings"=w533:refnum<vi>, "UI Data.Override.NG"=w527:string)
        n210 = property class="Str"(reference=w536, error in=w532, "Value"=w526) -> (error out=w535:errorcluster)  [unwired: 1 out]
        n211 = property class="Str"(reference=w534, error in=w532, "Value"=w528) -> (error out=w530:errorcluster)  [unwired: 1 out]
        n212 = property class="Str"(reference=w533, error in=w532, "Value"=w527) -> (error out=w529:errorcluster)  [unwired: 1 out]
        n213 = Merge Errors(w535, w530, w529) -> (w531:errorcluster)
        n214 = call <vilib>:"Add State(s) to Queue__JKI_lib_State_Machine.vi"("State(s) in (\"\")"=w540) -> ("States Out"=w539:string)  [unwired: 14 in]
      }
      frame "---------- Generate ----------" {
        n215 = call <vilib>:"Add State(s) to Queue__JKI_lib_State_Machine.vi"("State(s) in (\"\")"=w545) -> ("States Out"=w544:string)  [unwired: 14 in]
      }
      frame "Generate: Stop" {
        n216 = Unbundle By Name(w548) -> ("UDE Data.Stop UDE"=w550:refnum<user-event>)
        n217 = Generate User Event(user event=w550, event data cluster=TRUE ("event data"), error in=w552) -> (user event out=w546:refnum<user-event>, error out=w551:errorcluster)  [unwired: 1 in]
        n218 = Bundle By Name(cluster=w548, "UDE Data.Stop UDE"=w546) -> (w547:T23)
        n219 = call <vilib>:"Add State(s) to Queue__JKI_lib_State_Machine.vi"("State(s) in (\"\")"=w555) -> ("States Out"=w554:string)  [unwired: 14 in]
      }
      frame "Generate: Actions" {
        n220 = Unbundle By Name(w568) -> ("Actions"=w565:bool[], "Main App Cluster.FROM DATE"=w564:refnum<vi>, "Main App Cluster.TO DATE"=w563:refnum<vi>, "Main App Cluster.PLC NUMBER"=w562:refnum<vi>, "Main App Cluster.MODEL-Setting"=w561:refnum<vi>, "Main App Cluster.CUSTOMER PART NUMBER-Setting"=w560:refnum<vi>, "Main App Cluster.SUPPLIER CODE-Setting"=w559:refnum<vi>, "Main App Cluster.LH / RH"=w558:refnum<vi>, "Main App Cluster.SAVED MODEL"=w556:refnum<vi>, "Main App Cluster.SEQUENCE NUMBER-Settings"=w557:refnum<vi>, "UDE Data.Controller UDE"=w571:refnum<user-event>)
        n221 = Bundle By Name(cluster=T18 {"Actions"=[], "UI Elements Cluster"={"Application Name"=refnum, "Tab Control"=refnum, "Status"=refnum, "Version No"=refnum, "Result Table"=refnum, "PLC"=refnum, "Database"=refnum, "Printer"=refnum, "Scanner"=refnum, "SHIFT"=refnum, "OK"=refnum, "NG"=refnum, "TOTAL"=refnum, "SCANNED BARCODE"=refnum, " PRINTED BARCODE"=refnum, "PART NUMBER"=refnum, "PRODUCTION DATE"=refnum, "SUPPLIER CODE"=refnum, "SEQUENCE NUMBER"=refnum, "MODEL"=refnum, "Settings"=refnum, "Report"=refnum, "Report Table"=refnum, "Home"=refnum, "Export"=refnum, "Fetch"=refnum, "TO DATE"=refnum, "FROM DATE"=refnum, "Model Table"=refnum, "Traceablity Graph"=refnum, "Override Button"=refnum, "Load Button"=refnum, "Home Button-Setting"=refnum, "Delete Button"=refnum, "Update Button"=refnum, "Save Button"=refnum, "SEQUENCE NUMBER-Settings"=refnum, "PLC NUMBER"=refnum, "LH / RH"=refnum, "SUPPLIER CODE-Setting"=refnum, "CUSTOMER PART NUMBER-Setting"=refnum, "MODEL-Setting"=refnum, "SAVED MODEL"=refnum, "NG-Settings"=refnum, "OK-Settings"=refnum}, "Modbus Data"={"IP Address"="", "Timeout"=0, "Port [502]"=0, "isSimulation?"=FALSE, "Model Number"=0, "Read Modbus Register"={"Starting Address"=0, "Number of Inputs"=1}, "Individual Address"=[], "Model Changed?"=FALSE, "Models Table"=[], "Status?"=FALSE}, "Print Data"={"Print Button"=FALSE, "VISA resource name"="", "Status?"=FALSE, "Scan?"=FALSE}, "Scan Data"={"Scan Button"=FALSE, "Status?"=FALSE}} ("event data"), "Actions"=w565, "UI Elements Cluster.FROM DATE"=w564, "UI Elements Cluster.TO DATE"=w563, "UI Elements Cluster.PLC NUMBER"=w562, "UI Elements Cluster.MODEL-Setting"=w561, "UI Elements Cluster.CUSTOMER PART NUMBER-Setting"=w560, "UI Elements Cluster.SUPPLIER CODE-Setting"=w559, "UI Elements Cluster.LH / RH"=w558, "UI Elements Cluster.SAVED MODEL"=w556, "UI Elements Cluster.SEQUENCE NUMBER-Settings"=w557) -> (w569:T18)
        n222 = Generate User Event(user event=w571, event data cluster=w569, error in=w573) -> (user event out=w566:refnum<user-event>, error out=w572:errorcluster)  [unwired: 1 in]
        n223 = Bundle By Name(cluster=w568, "UDE Data.Controller UDE"=w566) -> (w567:T23)
        n224 = call <vilib>:"Add State(s) to Queue__JKI_lib_State_Machine.vi"("State(s) in (\"\")"=w576) -> ("States Out"=w575:string)  [unwired: 14 in]
      }
    }
  }
  "Error Out" <- w3
